vi "parsiranje.vi"(11 "Ulaz":string) -> (2 "Argument":string, 3 "Stanje":string)   [LabVIEW 2023]
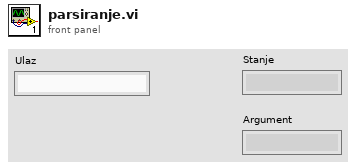
[diagram p1: front panel]
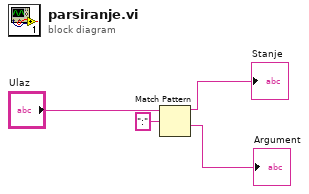
[diagram p0: block diagram]
diagram:
  n1 = Match Pattern(string="Ulaz", regular expression=":") -> (before substring=→"Stanje":string, after substring=→"Argument":string)  [unwired: 1 in, 2 out]
